vi "Set Selected Dye.vi"(8 "error in (no error)":errorcluster, 9 "Select Dye String":string, 10 "Selected Dye":i32=-1, 11 "Settings in":refnum<class "Settings.lvclass">) -> (0 "error out":errorcluster, 3 "Settings out":refnum<class "Settings.lvclass">)   [LabVIEW 2010, in "Settings.lvclass"]
uses:
  Settings.lvclass
  Settings.lvclass/Settings.ctl
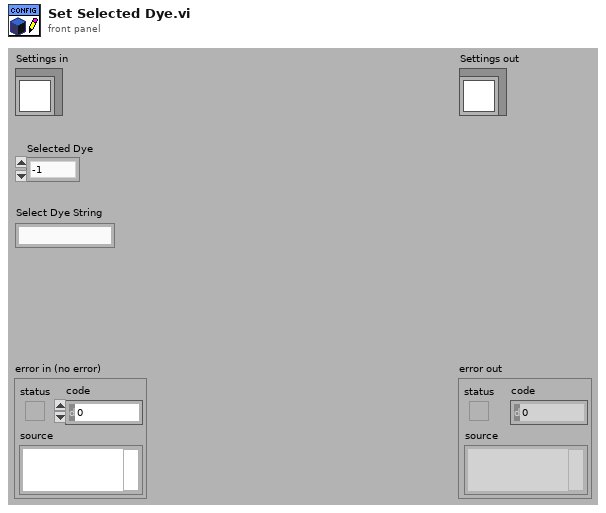
[diagram p1: front panel]
types:
  T1 = cluster{"Dye Name":string, "Pulse Sequence":cluster{"LED Name":string, "Pulse Length (s)":dbl, "Delay Before (s)":dbl, "Delay After (s)":dbl, "Trigger Camera":bool}[], "Emission Filter":i16, "Exposure (s)":dbl, "Yellow Select":bool, "# Pulses":i32}[]
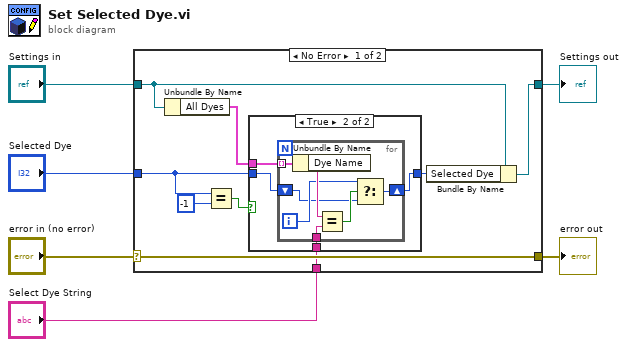
[diagram p0: block diagram]
diagram:
  n1 = case shown="No Error" "error in (no error)" {
    selector: "error in (no error)" -> [w15 w28]
    tunnel: [w15 w28] -> w5
    tunnel: [w14 w29] -> w3
    tunnel: "Settings in" -> [w9 w29]
    tunnel: "Selected Dye" -> [w11 _]
    tunnel: "Select Dye String" -> [w7 _]
    frame No Error {
      n2 = Unbundle By Name(w9) -> ("All Dyes"=w8:T1)
      n3 = Equal?(x=w11, y=-1) -> (x = y?=w12:bool)
      n4 = case shown="True" w12 {
        tunnel: w11 -> [w16 w19]
        tunnel: [w16 w18] -> w10
        tunnel: w8 -> [_ w20]
        tunnel: w7 -> [_ w17]
        frame False {
        }
        frame True {
          n5 = for {
            tunnel: w20 -> [w27] mode=indexing
            shift-right: [w23] -> w18
            shift-left: w19 -> [w21]
            tunnel: w17 -> [w25]
            i -> [w22]
            n6 = Unbundle By Name(w27) -> ("Dye Name"=w26:string)
            n7 = Equal?(x=w26, y=w25) -> (x = y?=w24:bool)
            n8 = Select(t=w22, s=w24, f=w21) -> (s? t:f=w23:i32)
          }
        }
      }
      n9 = Bundle By Name(cluster=w9, "Selected Dye"=w10) -> (w14:refnum<class "Settings.lvclass">)
    }
    frame Error {
    }
  }
  "error out" <- w5
  "Settings out" <- w3
